vi "notifierTest.vi"() -> ()   [LabVIEW 2020]
panel:
  out "number (0 to 1) 2":dbl
  out "number (0 to 1)":dbl
  in  "stop 2":bool
  in  "stop":bool
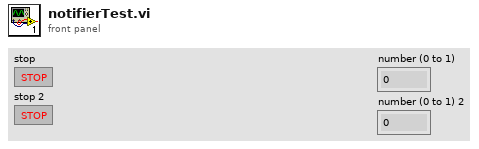
[diagram p1: front panel]
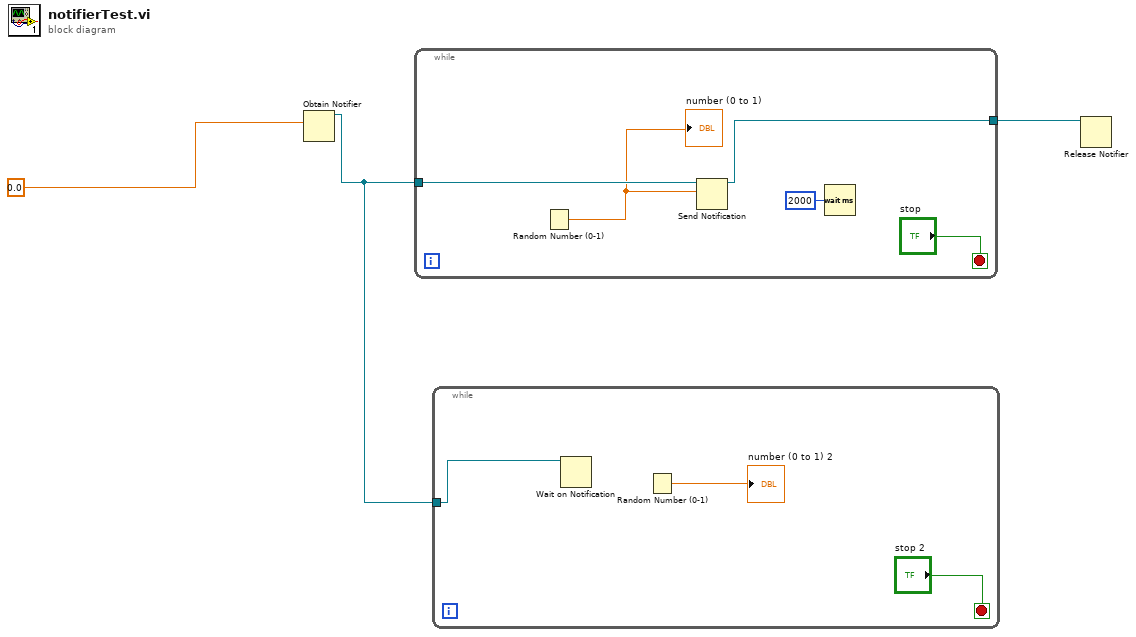
[diagram p0: block diagram]
diagram:
  n1 = Obtain Notifier(notification data type=0.0) -> (notifier out=w1:refnum<notifier>)  [unwired: 3 in, 2 out]
  n2 = while {
    tunnel: w1 -> [w7]
    tunnel: [w5] -> w2
    stop <- "stop" stop-if-true
    n3 = Random Number (0-1)() -> (number: 0 to 1=w6:dbl)
    "number (0 to 1)" <- w6
    n4 = Send Notification(notification=w6, notifier=w7) -> (notifier out=w5:refnum<notifier>)  [unwired: 1 in, 1 out]
    n5 = Wait (ms)(milliseconds to wait=u32 2000) -> ()  [unwired: 1 out]
  }
  n6 = while {
    tunnel: w1 -> [w9]
    stop <- "stop 2" stop-if-true
    n7 = Wait on Notification(notifier=w9) -> ()  [unwired: 3 in, 4 out]
    n8 = Random Number (0-1)() -> (number: 0 to 1=→"number (0 to 1) 2":dbl)
  }
  n9 = Release Notifier(notifier=w2) -> ()  [unwired: 2 in, 3 out]
